vi "close modules.vi"(11 "close FP?":bool) -> ()   [LabVIEW 2017]
doc: "SciScan 1.2 160622"
panel:
  out "Array 3":errorcluster[](array[cluster])
  out "Array 2":T1(array[cluster])
  out "Array":errorcluster[](array[cluster])
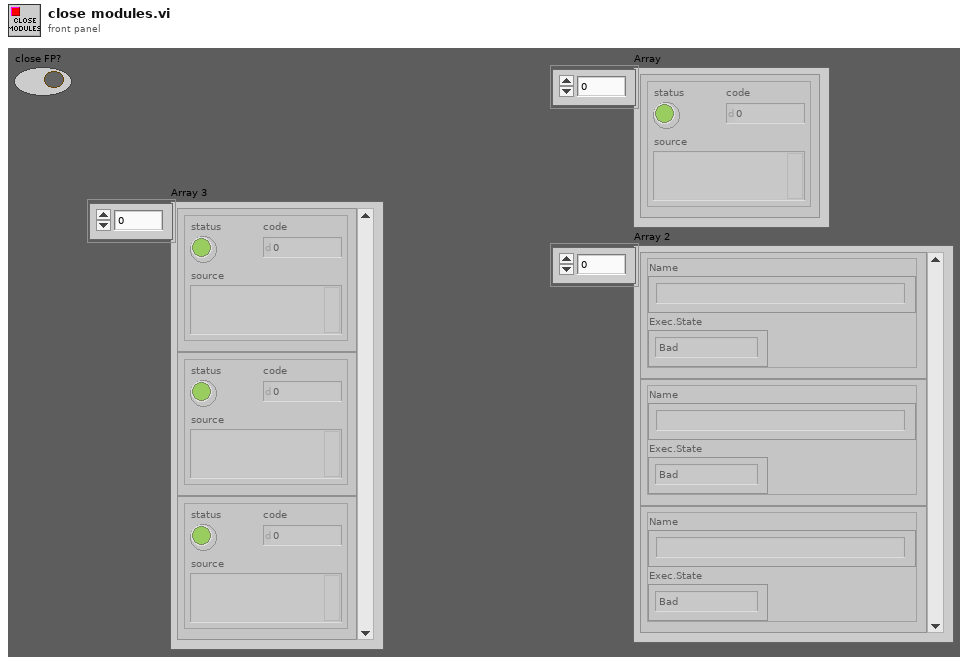
[diagram p1: front panel]
types:
  T1 = cluster{"Name":string, "Exec.State":enum32{"Bad", "Idle", "Run top level", "Running"}}[]
  T2 = enum32{"Bad", "Idle", "Run top level", "Running"}
  T3 = cluster{"Name":string, "Exec.State":enum32{"Bad", "Idle", "Run top level", "Running"}}
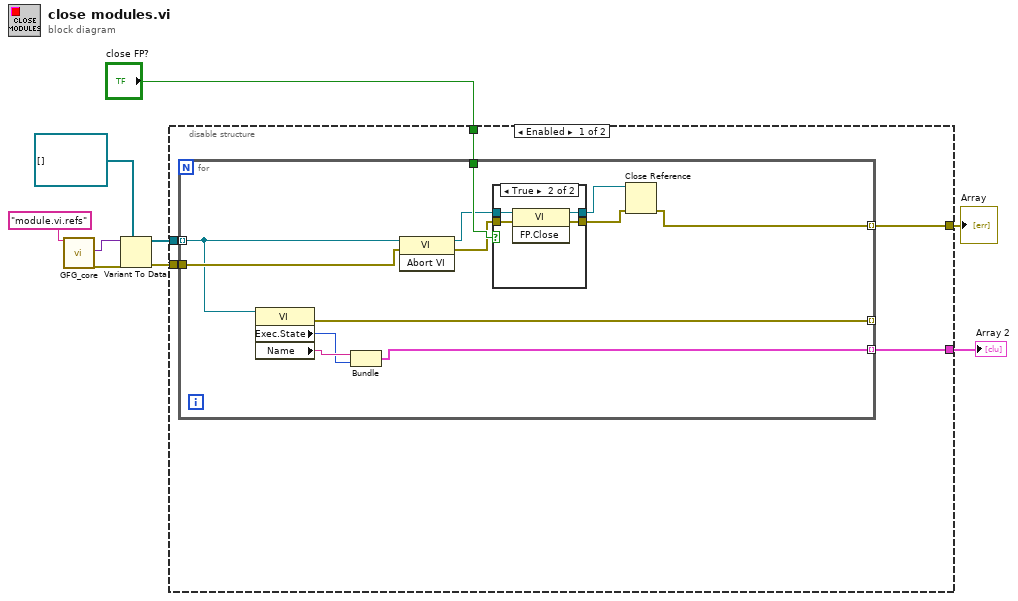
[diagram p0: block diagram]
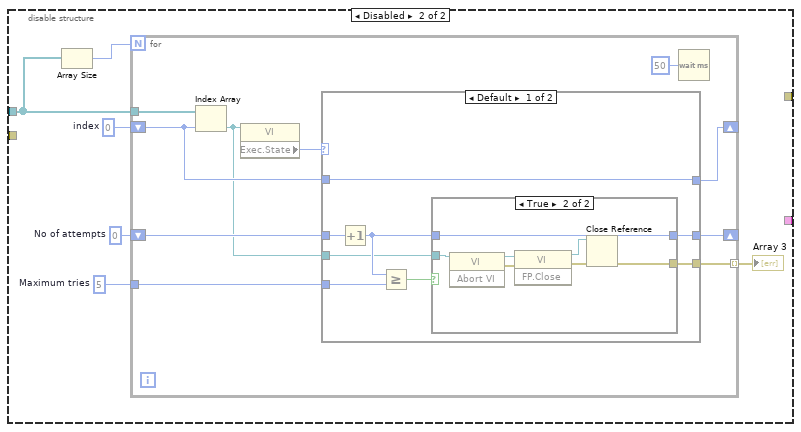
[diagram p3: hidden frame]
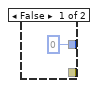
[diagram p4: hidden frame]
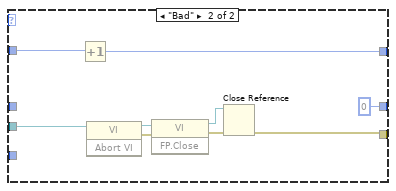
[diagram p5: hidden frame]
diagram:
  n1 = call "GFG_core.vi"("Variable Name in"="module.vi.refs") -> ("Variant Out"=w7:variant, "error out"=w8:errorcluster)  [unwired: 12 in, 5 out]
  n2 = Variant To Data(error in=w8, type=refnum<vi>[] [], Variant=w7) -> (data=w5:refnum<vi>[], error out=w4:errorcluster)
  n3 = disable-structure shown="Enabled" {
    disable-tunnel: w5 -> [w14 w38]
    disable-tunnel: w4 -> [w13 _]
    disable-tunnel: [w12 _] -> w3
    disable-tunnel: "close FP?" -> [w11 _]
    disable-tunnel: [w10 _] -> w1
    frame Enabled {
      n4 = for {
        tunnel: w14 -> [w19] mode=indexing
        tunnel: w13 -> [w23]
        tunnel: [w20] -> w12 mode=indexing
        tunnel: w11 -> [w26]
        tunnel: [w16] -> w10 mode=indexing
        tunnel: [w15] -> _ mode=indexing
        n5 = property class="VI"(reference=w19) -> (error out=w15:errorcluster, "Exec.State"=w17:T2, "Name"=w18:string)  [unwired: 1 in, 1 out]
        n6 = Bundle("Name"=w18, "Exec.State"=w17) -> (w16:T3)  [unwired: 1 in]
        n7 = invoke class="VI" method="Abort VI"(reference=w19, error in=w23) -> (reference out=w25:refnum<vi>, error out=w24:errorcluster)  [unwired: 1 in, 1 out]
        n8 = case shown="True" w26 {
          tunnel: w25 -> [w28 w32]
          tunnel: [w28 w31] -> w22
          tunnel: [w27 w30] -> w21
          tunnel: w24 -> [w27 w29]
          frame False {
          }
          frame True {
            n9 = invoke class="VI" method="FP.Close"(reference=w32, error in=w29) -> (reference out=w31:refnum<vi>, error out=w30:errorcluster)  [unwired: 1 in, 1 out]
          }
        }
        n10 = Close Reference(reference=w22, error in (no error)=w21) -> (error out=w20:errorcluster)
      }
    }
    frame Disabled {
      w34 = 5  # Maximum tries
      w35 = 0  # No of attempts
      w36 = 0  # index
      n11 = Array Size(array=w38) -> (size(s)=w37:i32)
      n12 = for {
        N: w37 -> [_]
        shift-right: [w45] -> _
        shift-left: w36 -> [w46]
        tunnel: w38 -> [w48]
        shift-right: [w41] -> _
        shift-left: w35 -> [w43]
        tunnel: w34 -> [w42]
        tunnel: [w39] -> w33 mode=indexing
        n13 = Index Array(array=w48, index=w46) -> (element=w40:refnum<vi>)
        n14 = property class="VI"(reference=w40) -> ("Exec.State"=w47:T2)  [unwired: 1 in, 2 out]
        n15 = case shown="Default" w47 {
          tunnel: w46 -> [w56 w73]
          tunnel: [w56 w72] -> w45
          tunnel: w43 -> [w55 _]
          tunnel: w42 -> [w54 _]
          tunnel: [w51 0] -> w41
          tunnel: w40 -> [w50 w66]
          tunnel: [w49 w65] -> w39
          frame Default {
            n16 = Increment(x=w55) -> (x+1=w52:i32)
            n17 = Greater Or Equal?(x=w52, y=w54) -> (x >= y?=w53:bool)
            n18 = case shown="True" w53 {
              tunnel: w52 -> [_ w64]
              tunnel: [0 w64] -> w51
              tunnel: w50 -> [_ w63]
              tunnel: [_ w59] -> w49
              frame False {
              }
              frame True {
                n19 = invoke class="VI" method="Abort VI"(reference=w63) -> (reference out=w62:refnum<vi>, error out=w58:errorcluster)  [unwired: 2 in, 1 out]
                n20 = invoke class="VI" method="FP.Close"(reference=w62, error in=w58) -> (reference out=w60:refnum<vi>, error out=w61:errorcluster)  [unwired: 1 in, 1 out]
                n21 = Close Reference(reference=w60, error in (no error)=w61) -> (error out=w59:errorcluster)
              }
            }
          }
          frame "Bad" {
            n22 = Increment(x=w73) -> (x+1=w72:i32)
            n23 = invoke class="VI" method="Abort VI"(reference=w66) -> (reference out=w70:refnum<vi>, error out=w67:errorcluster)  [unwired: 2 in, 1 out]
            n24 = invoke class="VI" method="FP.Close"(reference=w70, error in=w67) -> (reference out=w68:refnum<vi>, error out=w69:errorcluster)  [unwired: 1 in, 1 out]
            n25 = Close Reference(reference=w68, error in (no error)=w69) -> (error out=w65:errorcluster)
          }
        }
        n26 = Wait (ms)(milliseconds to wait=u32 50) -> ()  [unwired: 1 out]
      }
      "Array 3" <- w33
    }
  }
  "Array" <- w3
  "Array 2" <- w1
